vi "appendpayload.vi"(1 "jsontoappend":string, 2 "basejson":string) -> (0 "concatenated json string":string)   [LabVIEW 2016]
doc: "Append a json string to another one.\nDoes not check for duplicate fields."
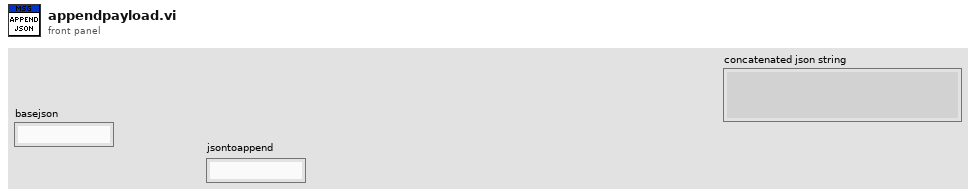
[diagram p1: front panel]
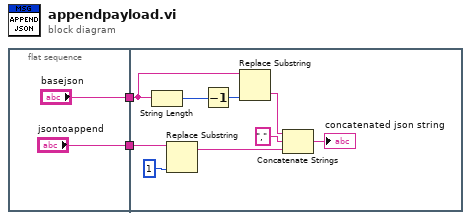
[diagram p0: block diagram]
diagram:
  n1 = flat-sequence {
    tunnel: ["basejson"] -> w2
    tunnel: ["jsontoappend"] -> w1
    tunnel: w2 -> [w12]
    tunnel: w1 -> [w10]
    frame #0 {
    }
    frame #1 {
      n2 = String Length(string=w12) -> (length=w13:i32)
      n3 = Replace Substring(2:1 ("length (len. of substring)"), 5:w10) -> (1:w5:string)  [unwired: 2 in, 1 out]
      n4 = Decrement(x=w13) -> (x-1=w8:i32)
      n5 = Replace Substring(2:w8, 5:w12) -> (0:w7:string)  [unwired: 2 in, 1 out]
      n6 = Concatenate Strings(w7, ",", w5) -> (→"concatenated json string":string)
    }
  }
